vi "SparkMAXConfigLimitSwitch.vi"(5 "Enabled?":bool, 6 "Error (in)":errorcluster, 7 "Polarity":T6, 8 "fwd/rev limit":T7, 9 "Device Reference (in)":T1) -> (0 "Error (out)":errorcluster, 3 "Device Reference (out)":T1={"DeviceStatus"={"status"=FALSE, "code"=0, "source"=""}, "Type"=enum."PWM", "PWM"={"PWM Channel"=enum."Invalid", "DeadBand"={"Name"="", "maxPositivePwm"=0, "minPositivePwm"=0, "centerPwm"=0, "maxNegativePwm"=0, "minNegativePwm"=0, "angularRange"=0}}, "CAN"={"Device Number"=0, "SetOutput VI Ref"=variant, "GetOutput VI Ref"=variant, "Enable VI Ref"=variant, "Disable VI Ref"=variant, "Data"=variant}, "Invert"=FALSE, "DIO PWM"={"PWM \"Enable\" Channel"=enum."Invalid", "DIOChannel"=enum."Invalid", "PWM Rate"=0.0}})   [LabVIEW 2023]
doc: "Wrapper for commanding the power of a Talon FX motor controller. Supports voltage and safety interlock. Also supports the standard actuator testing interface and and the only sending new values on change."
uses:
  <vilib>/Rock Robotics/WPI/MotorControl/WPI_MotorControlDeviceRef.ctl
  <vilib>/Rock Robotics/WPI/MotorControl/WPI_MotorControlType.ctl
  <vilib>/Rock Robotics/SystemInterfaces/DIO/FPGA_DIOPWMChannel.ctl
  <vilib>/Rock Robotics/WPI/PWM/WPI_PWMDeadband.ctl
  <vilib>/Rock Robotics/SystemInterfaces/DIO/FPGA_DIOChannel.ctl
  a6b6150a-d8ea-4c9f-aab9-93d54f9e21f2.vi
  <vilib>/Rock Robotics/WPI/ThirdParty/REV Robotics/REVLib/Typedef/Spark MAX Limit Direction.ctl
  <vilib>/Rock Robotics/WPI/ThirdParty/REV Robotics/REVLib/Typedef/Spark MAX Limit Switch Polarity.ctl
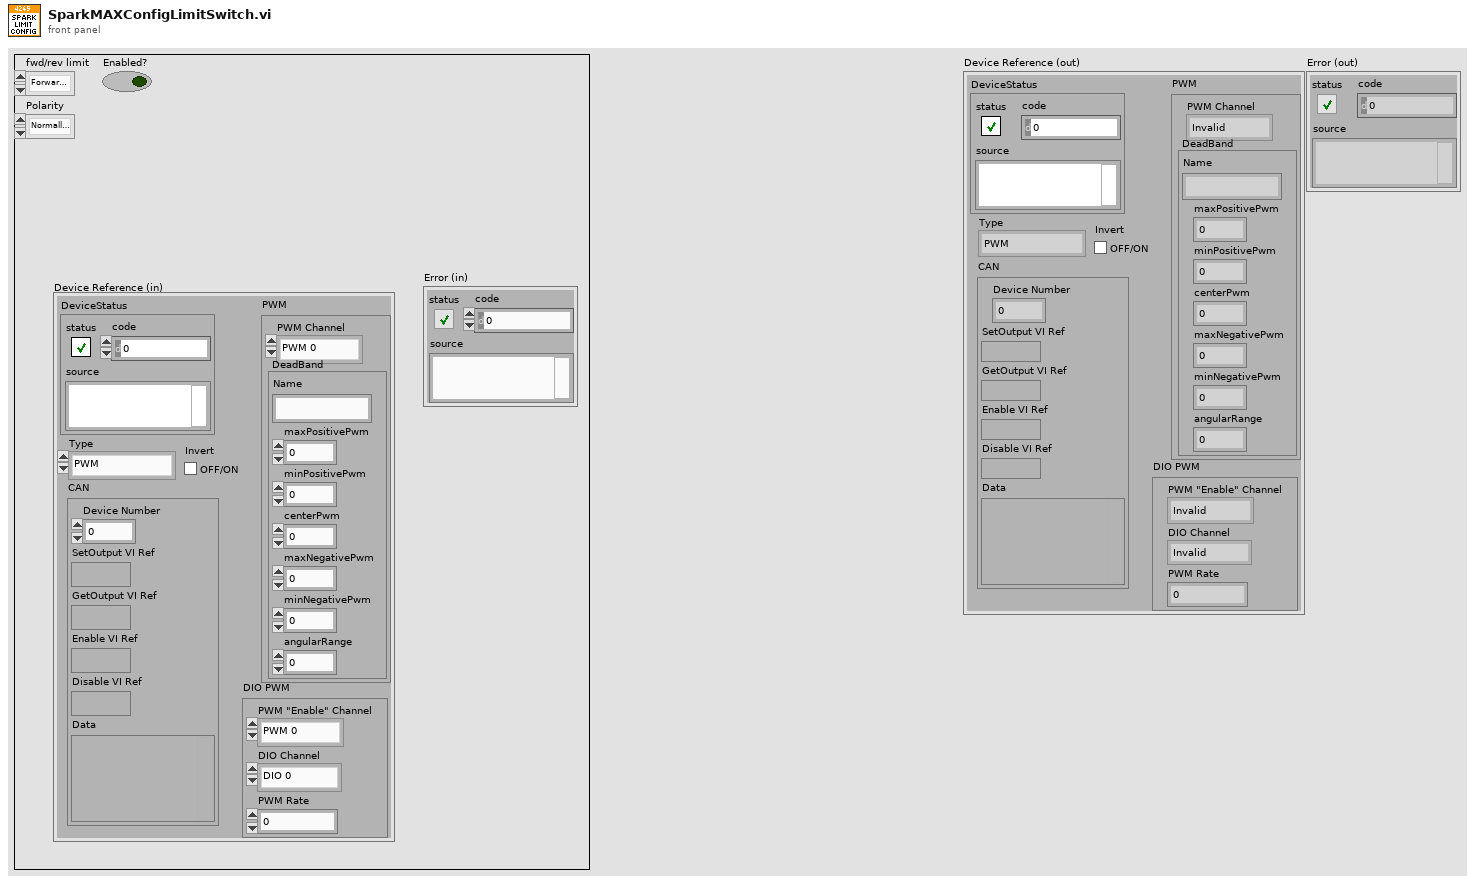
[diagram p1: front panel]
types:
  T1 = typedef "WPI_MotorControlDeviceRef.ctl" = cluster{"DeviceStatus":errorcluster, "Type":T2, "PWM":cluster{"PWM Channel":T3, "DeadBand":T4}, "CAN":cluster{"Device Number":u8, "SetOutput VI Ref":variant, "GetOutput VI Ref":variant, "Enable VI Ref":variant, "Disable VI Ref":variant, "Data":variant}, "Invert":bool, "DIO PWM":cluster{"PWM \"Enable\" Channel":T3, "DIOChannel":T5, "PWM Rate":dbl}}
  T2 = typedef "WPI_MotorControlType.ctl" = enum16{"PWM", "CAN", "DIO PWM"}
  T3 = typedef "FPGA_DIOPWMChannel.ctl" = enum8{"PWM 0", "PWM 1", "PWM 2", "PWM 3", "PWM 4", "PWM 5", "PWM 6", "PWM 7", "PWM 8", "PWM 9", "PWM MXP 0", "PWM MXP 1", "PWM MXP 2", "PWM MXP 3", "PWM MXP 4", "PWM MXP 5", "PWM MXP 6", "PWM MXP 7", "PWM MXP 8", "PWM MXP 9", "Invalid"}
  T4 = typedef "WPI_PWMDeadband.ctl" = cluster{"Name":string, "maxPositivePwm":i32, "minPositivePwm":i32, "centerPwm":i32, "maxNegativePwm":i32, "minNegativePwm":i32, "angularRange":u16}
  T5 = typedef "FPGA_DIOChannel.ctl" = enum8{"DIO 0", "DIO 1", "DIO 2", "DIO 3", "DIO 4", "DIO 5", "DIO 6", "DIO 7", "DIO 8", "DIO 9", "DIO MXP 0", "DIO MXP 1", "DIO MXP 2", "DIO MXP 3", "DIO MXP 4", "DIO MXP 5", "DIO MXP 6", "DIO MXP 7", "DIO MXP 8", "DIO MXP 9", "DIO MXP 10", "DIO MXP 11", "DIO MXP 12", "DIO MXP 13", "DIO MXP 14", "DIO MXP 15", "SPI Port CS1", "SPI Port CS2", "SPI Port CS3", "SPI Port MISO", "SPI Port MOSI", "Invalid"}
  T6 = typedef "Spark MAX Limit Switch Polarity.ctl" = enum16{"Normally Open", "Normally Closed"}
  T7 = typedef "Spark MAX Limit Direction.ctl" = enum16{"Forward Limit", "Reverse Limit"}
  T8 = cluster{"Enabled?":bool, "Device Reference (in)":T1, "Error (in)":errorcluster, "fwd/rev limit":T7, "Polarity":T6}
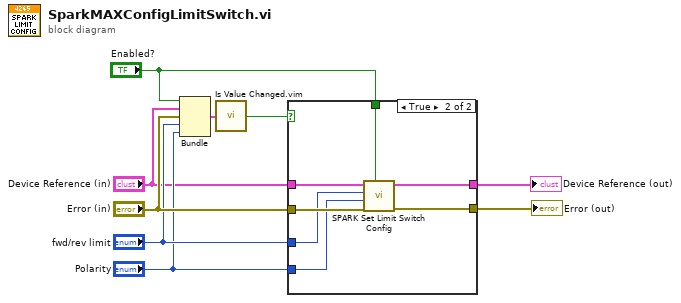
[diagram p0: block diagram]
diagram:
  n1 = Bundle("Enabled?"="Enabled?", "Device Reference (in)"="Device Reference (in)", "Error (in)"="Error (in)", "fwd/rev limit"="fwd/rev limit", "Polarity"="Polarity") -> (w5:T8)  [unwired: 1 in]
  n2 = call "Is Value Changed.vim"("value"=w5) -> ("changed or first call?"=w4:bool)
  n3 = case shown="True" w4 {
    tunnel: "Device Reference (in)" -> [w11 w18]
    tunnel: "Error (in)" -> [w10 w17]
    tunnel: "fwd/rev limit" -> [_ w16]
    tunnel: "Polarity" -> [_ w15]
    tunnel: "Enabled?" -> [_ w14]
    tunnel: [w11 w13] -> w3
    tunnel: [w10 w12] -> w2
    frame False {
    }
    frame True {
      n4 = call <vilib>:"SPARK Set Limit Switch Config.vi"("Enabled? (T)"=w14, "error in (no error)"=w17, "Polarity (Normally Open)"=w15, "Limit Switch"=w16, "MotorControlDeviceRef in"=w18) -> ("error out"=w12:errorcluster, "MotorControlDeviceRef out"=w13:T1)  [unwired: 5 in]
    }
  }
  "Device Reference (out)" <- w3
  "Error (out)" <- w2
